vi "Initialize Stock Menu Items.vi"(8 "error in (no error)":errorcluster, 10 "Menu in":refnum<k9>, 11 "Code String in":refnum<class "Code String.lvclass">) -> (0 "error out":errorcluster, 2 "Menu out":refnum<k9>, 3 "Code String out":refnum<class "Code String.lvclass">)   [LabVIEW 2016, in "Code String.lvclass"]
doc: "Initializes the base context <b>Menu</b> in the <b>Code String</b> UI.\n--------------------\nCopyright (c) 2019 Analog Devices, Inc. All rights reserved.\n\nRedistribution and use in source and binary forms, with or without modification,\nare permitted provided that the following conditions are met:\n - Redistributions of source code must retain the above copyright notice, this\n list of conditions and the following disclaimer.\n - Redistributions in binary form must reproduce the above copyright notice,\n this list of conditions and the following disclaimer in the documentation\n and/or other materials provided with the distribution.\n - Modified versions of the software must be conspicuously marked as such.\n - This software is licensed solely and exclusively for use with\n processors/products manufactured by or for Analog Devices, Inc.\n - This software may not be combined or merged with other code in any manner\n that would cause the software to become subject to terms and conditions\n which differ from those listed here.\n - Neither the name of Analog Devices, Inc. nor the names of its contributors\n may be used to endorse or promote products derived from this software\n without specific prior written permission.\n - The use of this software may or may not infringe the patent rights of one or\n more patent holders. This license does not release you from the requirement\n that you obtain separate licenses from these patent holders to use this\n software.\n\nTHIS SOFTWARE IS PROVIDED BY ANALOG DEVICES, INC. AND CONTRIBUTORS \"AS IS\" AND\nANY EXPRESS OR IMPLIED WARRANTIES, INCLUDING, BUT NOT LIMITED TO,\nNON-INFRINGEMENT, TITLE, MERCHANTABILITY AND FITNESS FOR A PARTICULAR PURPOSE\nARE DISCLAIMED. IN NO EVENT SHALL ANALOG DEVICES, INC. OR CONTRIBUTORS BE LIABLE\nFOR ANY DIRECT, INDIRECT, INCIDENTAL, SPECIAL, EXEMPLARY, PUNITIVE OR\nCONSEQUENTIAL DAMAGES (INCLUDING, BUT NOT LIMITED TO, DAMAGES ARISING OUT OF\nCLAIMS OF INTELLECTUAL PROPERTY RIGHTS INFRINGEMENT; PROCUREMENT OF SUBSTITUTE\nGOODS OR SERVICES; LOSS OF USE, DATA, OR PROFITS; OR BUSINESS INTERRUPTION)\nHOWEVER CAUSED AND ON ANY THEORY OF LIABILITY, WHETHER IN CONTRACT, STRICT\nLIABILITY, OR TORT (INCLUDING NEGLIGENCE OR OTHERWISE) ARISING IN ANY WAY OUT OF\nTHE USE OF THIS SOFTWARE, EVEN IF ADVISED OF THE POSSIBILITY OF SUCH DAMAGE.\n\n2019-01-10-7CBSD SLA"
uses:
  Code String.lvclass
  Properties/Read Completion.vi
  Properties/Read Editable.vi
panel:
  # "Copyright (c) 2019 Analog Devices, Inc.  All rights reserved.\n\nRedistribution and use in source and binary forms, with or without modification,\nare permitted provided that the following conditions are met:\n  - Redistributions of source code must retain the above copyright notice, this\n    list of conditions and the following disclaimer.\n  - Redistributions in binary form must reproduce the above copyright notice,\n    this list of conditions and the following disclaimer in the documentation\n    and/or other materials provided with the distribution.\n  - Modified versions of the software must be conspicuously marked as such.\n  - This software is licensed solely and exclusively for use with\n    processors/products manufactured by or for Analog Devices, Inc.\n  - This software may not be combined or merged with other code in any manner\n    that would cause the software to become subject to terms and conditions\n    which differ from those listed here.\n  - Neither the name of Analog Devices, Inc. nor the names of its contributors\n    may be used to endorse or promote products derived from this software\n    without specific prior written permission.\n  - The use of this software may or may not infringe the patent rights of one or\n    more patent holders.  This license does not release you from the requirement\n    that you obtain separate licenses from these patent holders to use this\n    software.\n\nTHIS SOFTWARE IS PROVIDED BY ANALOG DEVICES, INC. AND CONTRIBUTORS \"AS IS\" AND\nANY EXPRESS OR IMPLIED WARRANTIES, INCLUDING, BUT NOT LIMITED TO,\nNON-INFRINGEMENT, TITLE, MERCHANTABILITY AND FITNESS FOR A PARTICULAR PURPOSE\nARE DISCLAIMED. IN NO EVENT SHALL ANALOG DEVICES, INC. OR CONTRIBUTORS BE LIABLE\nFOR ANY DIRECT, INDIRECT, INCIDENTAL, SPECIAL, EXEMPLARY, PUNITIVE OR\nCONSEQUENTIAL DAMAGES (INCLUDING, BUT NOT LIMITED TO, DAMAGES ARISING OUT OF\nCLAIMS OF INTELLECTUAL PROPERTY RIGHTS INFRINGEMENT; PROCUREMENT OF SUBSTITUTE\nGOODS OR SERVICES; LOSS OF USE, DATA, OR PROFITS; OR BUSINESS INTERRUPTION)\nHOWEVER CAUSED AND ON ANY THEORY OF LIABILITY, WHETHER IN CONTRACT, STRICT\nLIABILITY, OR TORT (INCLUDING NEGLIGENCE OR OTHERWISE) ARISING IN ANY WAY OUT OF\nTHE USE OF THIS SOFTWARE, EVEN IF ADVISED OF THE POSSIBILITY OF SUCH DAMAGE.\n\n2019-01-10-7CBSD SLA"
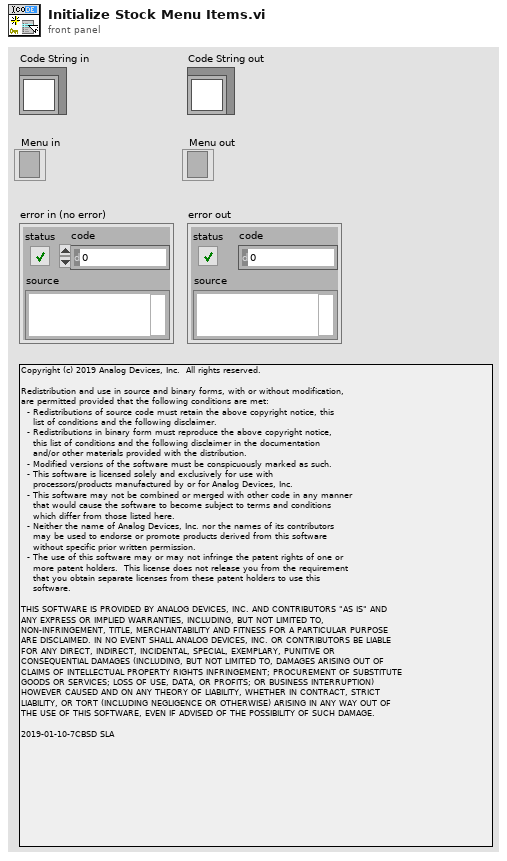
[diagram p1: front panel]
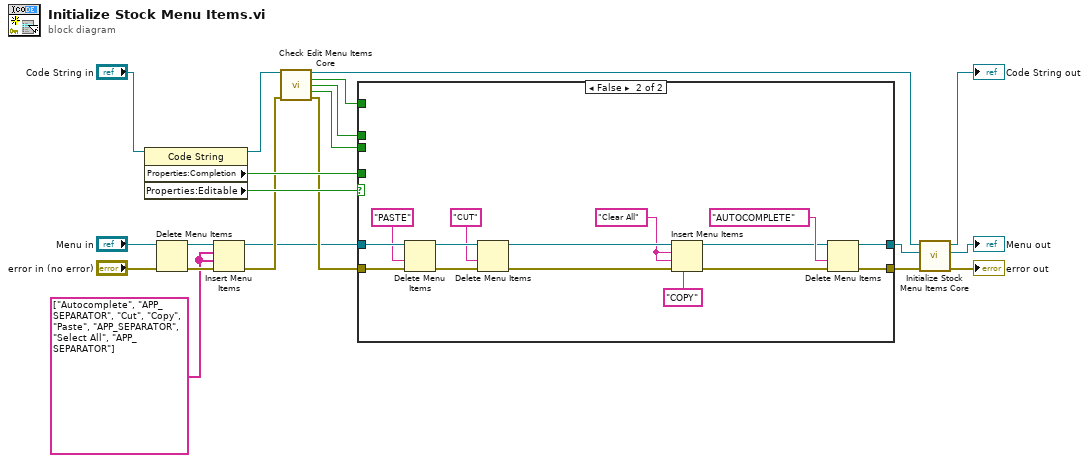
[diagram p0: block diagram]
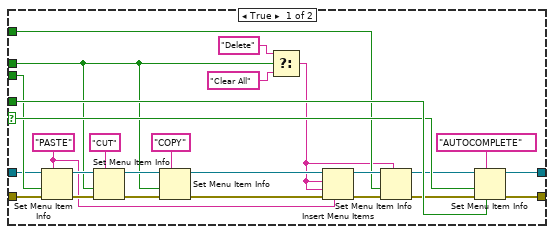
[diagram p2: hidden frame]
diagram:
  w13 = string[] ["Autocomplete", "APP_SEPARATOR", "Cut", "Copy", "Paste", "APP_SEPARATOR", "Select All", "APP_SEPARATOR"]
  n1 = property class="Code String"(reference="Code String in") -> (reference out=w11:refnum<class "Code String.lvclass">, "Properties:Completion"=w18:bool, "Properties:Editable"=w19:bool)  [unwired: 1 in, 1 out]
  n2 = Delete Menu Items(6:"error in (no error)", 9:"Menu in") -> (0:w16:errorcluster, 3:w14:refnum<k9>)  [unwired: 2 in]
  n3 = Insert Menu Items(6:w16, 7:w13, 8:w13, 9:w14) -> (0:w10:errorcluster, 3:w1:refnum<k9>)  [unwired: 2 in, 1 out]
  n4 = call-dynamic "Check Edit Menu Items Core.vi"("Code String in"=w11, "error in (no error)"=w10) -> ("Code String out"=w12:refnum<class "Code String.lvclass">, "Can Delete"=w3:bool, "Can Copy/Cut"=w4:bool, "Can Paste"=w9:bool, "error out"=w2:errorcluster)  [unwired: 9 in]
  n5 = case shown="False" w19 {
    selector: w19 -> [w41 _]
    tunnel: [w37 w62] -> w21
    tunnel: w18 -> [w47 _]
    tunnel: [w38 w57] -> w8
    tunnel: w9 -> [w40 _]
    tunnel: w4 -> [w34 _]
    tunnel: w3 -> [w25 _]
    tunnel: w2 -> [w30 w56]
    tunnel: w1 -> [w29 w55]
    frame True {
      w22 = "PASTE" ("item tag")
      n6 = Set Menu Item Info(7:w22, 8:w30, 9:w40, 11:w29) -> (0:w45:errorcluster, 3:w44:refnum<k9>)  [unwired: 3 in]
      n7 = Set Menu Item Info(7:"CUT" ("item tag"), 8:w45, 9:w34, 11:w44) -> (0:w42:errorcluster, 3:w39:refnum<k9>)  [unwired: 3 in]
      n8 = Set Menu Item Info(7:"COPY" ("item tag"), 8:w42, 9:w34, 11:w39) -> (0:w31:errorcluster, 3:w33:refnum<k9>)  [unwired: 3 in]
      n9 = Select(t="Delete", s=w34, f="Clear All") -> (s? t:f=w24:string)
      n10 = Insert Menu Items(4:w22, 6:w31, 7:w24, 8:w24, 9:w33) -> (0:w32:errorcluster, 3:w27:refnum<k9>)  [unwired: 1 in, 1 out]
      n11 = Set Menu Item Info(7:w24, 8:w32, 9:w25, 11:w27) -> (0:w28:errorcluster, 3:w26:refnum<k9>)  [unwired: 3 in]
      n12 = Set Menu Item Info(6:w47, 7:"AUTOCOMPLETE" ("item tag"), 8:w28, 9:w41, 11:w26) -> (0:w37:errorcluster, 3:w38:refnum<k9>)  [unwired: 2 in]
    }
    frame False {
      w49 = "Clear All" ("item name")
      n13 = Delete Menu Items(6:w56, 7:"PASTE" ("item tag"), 9:w55) -> (0:w61:errorcluster, 3:w60:refnum<k9>)  [unwired: 1 in]
      n14 = Delete Menu Items(6:w61, 7:"CUT" ("item tag"), 9:w60) -> (0:w53:errorcluster, 3:w54:refnum<k9>)  [unwired: 1 in]
      n15 = Insert Menu Items(4:"COPY" ("after item"), 6:w53, 7:w49, 8:w49, 9:w54) -> (0:w51:errorcluster, 3:w52:refnum<k9>)  [unwired: 1 in, 1 out]
      n16 = Delete Menu Items(6:w51, 7:"AUTOCOMPLETE" ("item tag"), 9:w52) -> (0:w62:errorcluster, 3:w57:refnum<k9>)  [unwired: 1 in]
    }
  }
  n17 = call-dynamic "Initialize Stock Menu Items Core.vi"("error in (no error)"=w21, "Menu in"=w8, "Code String in"=w12) -> ("error out"=→"error out":errorcluster, "Menu out"=→"Menu out":refnum<k9>, "Code String out"=→"Code String out":refnum<class "Code String.lvclass">)  [unwired: 6 in]
